vi "Module_ENG_TCPServer.vi"(8 "error in (no error)":errorcluster, 9 "Module ID (-1: Do not Address)":i32=-1, 10 "Wait on Module(s) (\"\": none)":string) -> (0 "error out":errorcluster)   [LabVIEW 2019, in "Module_ENG_TCPServer.lvclass"]
doc: "created using\nJSMA Module Template - ENGINE Class 0.2.1.12\nRob Humfeld - Jet Engineering\nCopyright (c) 2020, Jet Engineering"
uses:
  Module_ENG_TCPServer.lvclass
  <userlib>/Jet Engineering/JET_QSM/Code/Private/JET_QSM - Add State to Front [String API].vi
  Private/Module_ENG_TCPServer_jMsgTxList STYP.ctl
  Private/Module_ENG_TCPServer_jMsgRxList STYP.ctl
  <userlib>/Jet Engineering/JET_QSM/Code/Private/JET_QSM_InvalidOption STYP.ctl
  <userlib>/Jet Engineering/JET_QSM/Code/Private/JET_QSM - Add State [String API].vi
  Private/Module_ENG_TCPServer_EngineStatus STYP.ctl
  Private/Module_ENG_TCPServer_LocalData STYP.ctl
  <userlib>/Jet Engineering/JSMA/Libraries/jMsg_CORE/jMsg_JSMA_ModuleOnline/jMsg_JSMA_ModuleOnline.lvclass
  <userlib>/Jet Engineering/JSMA/Libraries/jMsg_CORE/jMsg_JSMA_ApplicationShutdown/jMsg_JSMA_ApplicationShutdown.lvclass
  <userlib>/Jet Engineering/JSMA/Libraries/jModule Class/jModule.lvclass
  Shared/TCP/jMsgs/jMsg_TCPMessage_Receive/jMsg_TCPMessage_Receive.lvclass
  Shared/TCP/jMsgs/jMsg_TCPMessage_Send/jMsg_TCPMessage_Send.lvclass
  <userlib>/Jet Engineering/JSMA/Libraries/jMsg Class/jMsg.lvclass
  Shared/TCP/jMsgs/jMsg_TCPAcceptor_NewConnection/jMsg_TCPAcceptor_NewConnection.lvclass
  labview_multiplayer_snake_personal/Main Codeline/Software/Code/Shared/TCPReceiver/TCPReceiver.lvclass
  Shared/TCP/TCPPacket/TCPPacket.lvclass
  Shared/TCP/jMsgs/jMsg_TCPServer_Status/jMsg_TCPServer_Status.lvclass
  labview_multiplayer_snake_personal/Main Codeline/Software/Code/Shared/JSONPacket/JSONPacket.lvclass
  C:/Program Files/National Instruments/LabVIEW 2019/user.lib/Jet Engineering/JSMA/Libraries/jModule Class/jModule.lvclass
  C:/projects/labview_multiplayer_snake_personal/Main Codeline/Software/Code/Shared/TCPPacket/TCPPacket.lvclass
  C:/Program Files/National Instruments/LabVIEW 2019/user.lib/Jet Engineering/JSMA/Libraries/jMsg Class/jMsg.lvclass
  <userlib>/Jet Engineering/JSMA/Libraries/jModule Class/Typedefs/jModule_TimerType STYP.ctl
  <userlib>/Jet Engineering/JSMA/Libraries/jModule Class/Typedefs/jModule_TimerConfig STYP.ctl
panel:
  out "Rx jMsg Subscriptions":string[](array[string])
  out "Timer Configuration":T1 {"Expiration Time" format="%<%.3X>T"}
  out "jModule Name":string
  out "iter":i32
  out "Latency, sec.":dbl
  out "RxTime":timestamp format="%<%H:%M:%S%3u>T"
  out "Last Rx Message":string
  out "Recent states before Error (with tick counts)":string
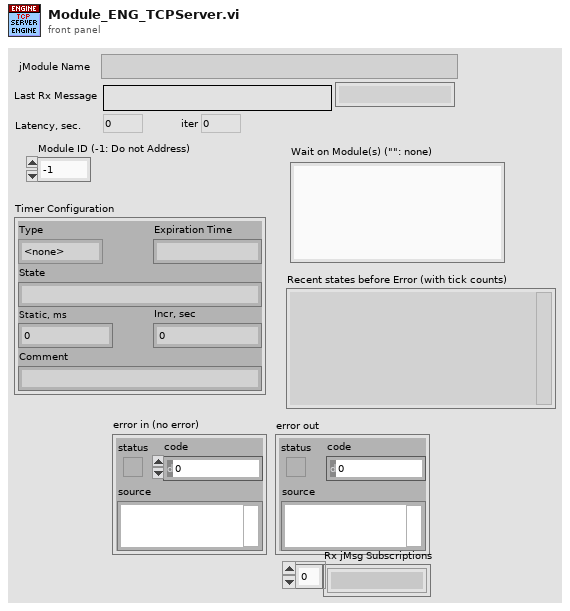
[diagram p1: front panel]
types:
  T1 = typedef "JSMA API.lvlib/jModule.lvclass/jModule_TimerConfig STYP.ctl" = cluster{"Type":T2, "Expiration Time":timestamp, "State":string, "Static, ms":i32, "Incr, sec":dbl, "Comment":string}
  T2 = typedef "JSMA API.lvlib/jModule.lvclass/jModule_TimerType STYP.ctl" = enum16{"<none>", "Static", "Countdown", "Periodic"}
  T3 = typedef "JET_QSM_InvalidOption STYP.ctl" = enum16{"Ignore", "Dialog", "Error"}
  T4 = cluster{"Connection ID":refnum<k5>, "TCPReceiver":refnum<class "TCPReceiver.lvclass">}[]
  T5 = typedef "Module_ENG_TCPServer.lvclass/Module_ENG_TCPServer_LocalData STYP.ctl" = cluster{"VI":cluster{"error":errorcluster, "isExiting?":bool}, "EngineStatus":T6}
  T6 = typedef "Module_ENG_TCPServer.lvclass/Module_ENG_TCPServer_EngineStatus STYP.ctl" = cluster{"Connections":cluster{"Connection ID":refnum<k5>, "TCPReceiver":refnum<class "TCPReceiver.lvclass">}[]}
  T7 = typedef "Module_ENG_TCPServer.lvclass/Module_ENG_TCPServer_jMsgRxList STYP.ctl" = cluster{"<placeholder>":refnum<class "jMsg_JSMA_ApplicationShutdown.lvclass">, "jMsg_TCPMessage_Send":refnum<class "jMsg_TCPMessage_Send.lvclass">, "jMsg_TCPAcceptor_NewConnection":refnum<class "jMsg_TCPAcceptor_NewConnection.lvclass">}
  T8 = typedef "Module_ENG_TCPServer.lvclass/Module_ENG_TCPServer_jMsgTxList STYP.ctl" = cluster{"<placeholder>":refnum<class "jMsg_JSMA_ModuleOnline.lvclass">, "jMsg_TCPMessage_Receive":refnum<class "jMsg_TCPMessage_Receive.lvclass">, "jMsg_TCPServer_Status":refnum<class "jMsg_TCPServer_Status.lvclass">}
  T9 = typedef "JET_QSM_Refnum STYP.ctl" = cluster{"state":cluster{"queue":refnum<queue>, "idle":string, "error":string, "STOP":string}, "debug":cluster{"enabled?":bool, "queue":refnum<queue>}, "Invalid.option":T3, "QSM.Name":string}
  T10 = typedef "JET_QSM_Element STYP.ctl" = cluster{"state":string, "data":variant, "comment":string}
  T11 = cluster{"Connection ID":refnum<k5>, "TCPReceiver out":refnum<class "TCPReceiver.lvclass">}
  T12 = cluster{"Connection ID":refnum<k5>, "TCPReceiver out":refnum<class "TCPReceiver.lvclass">}[]
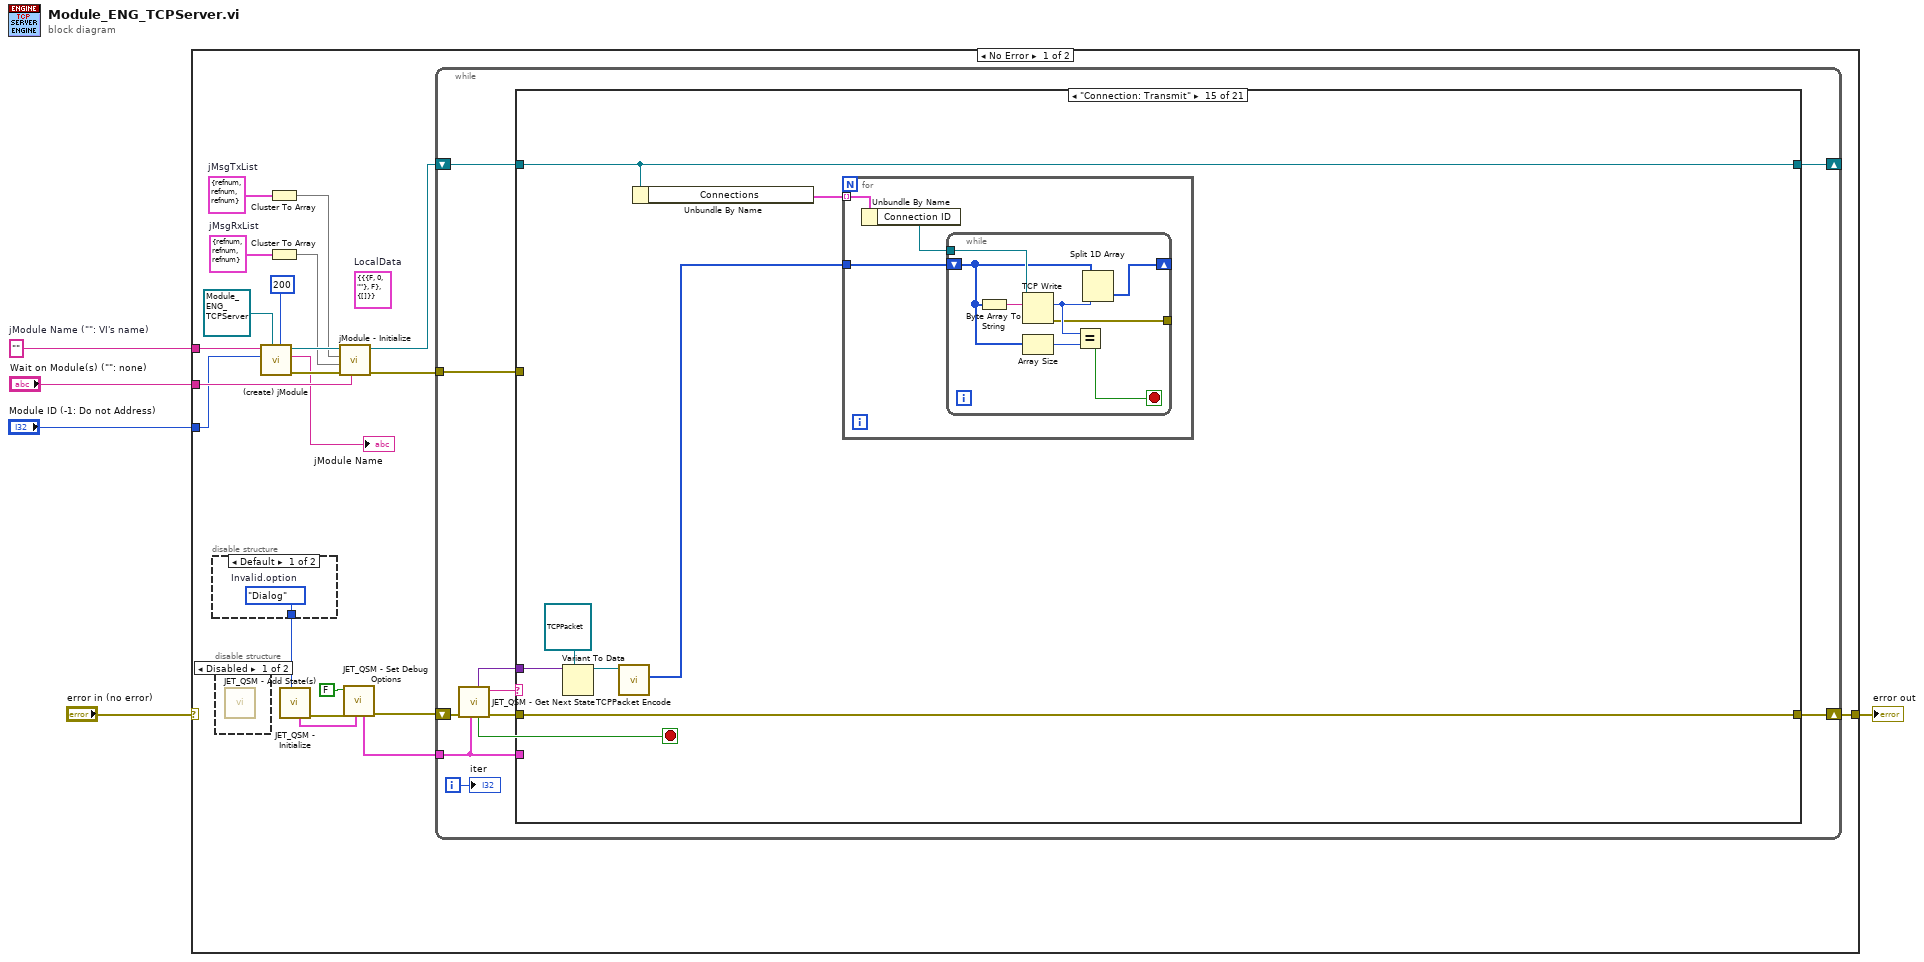
[diagram p0: block diagram]
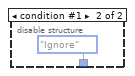
[diagram p3: hidden frame]
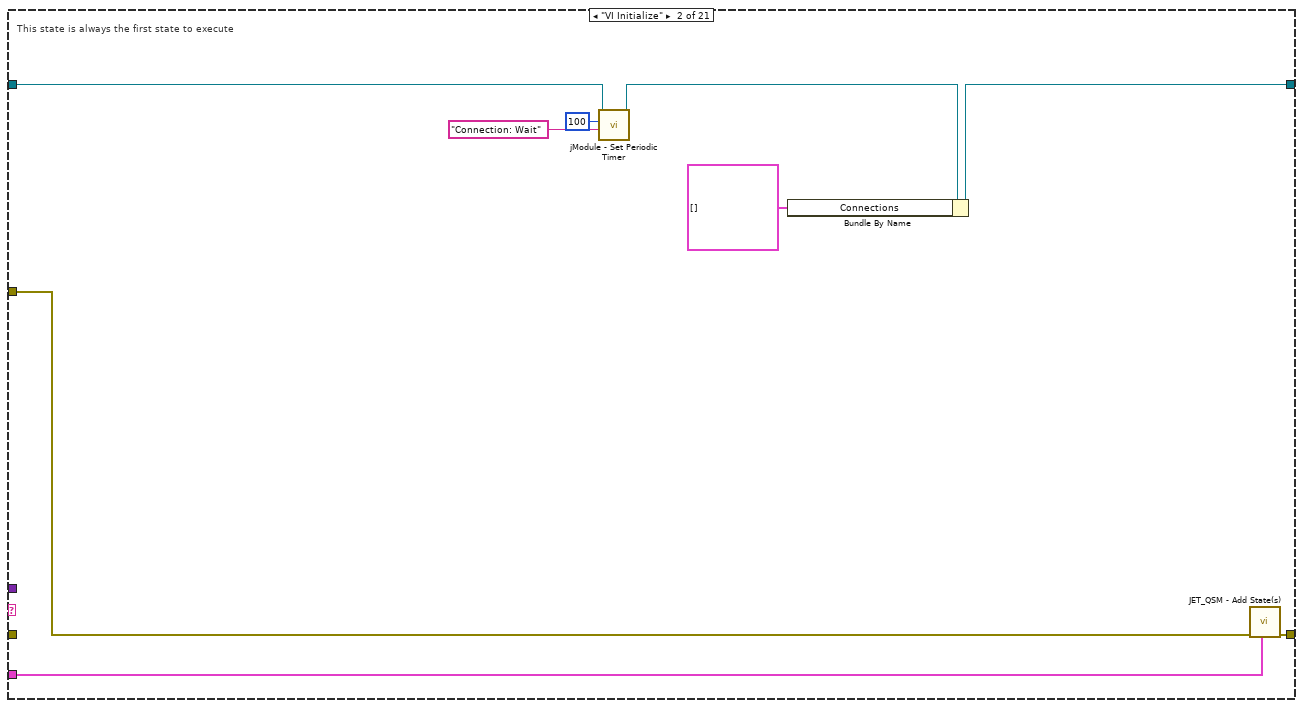
[diagram p5: hidden frame]
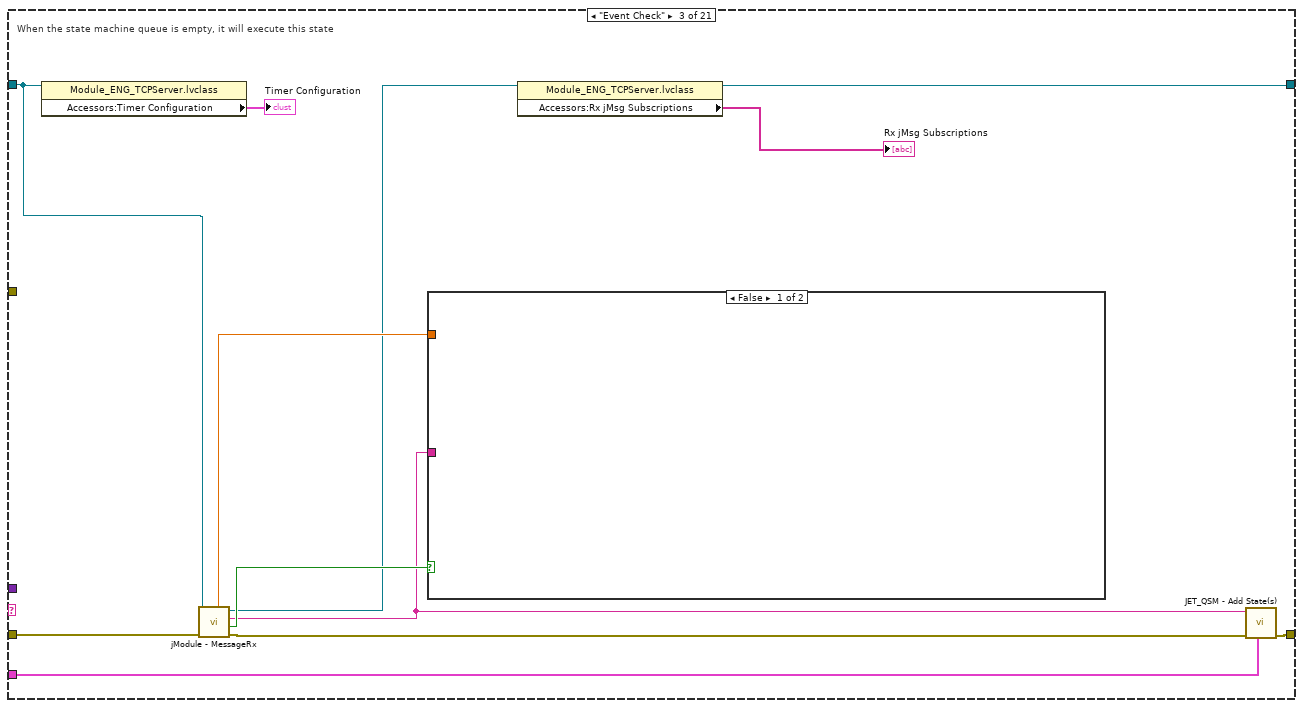
[diagram p6: hidden frame]
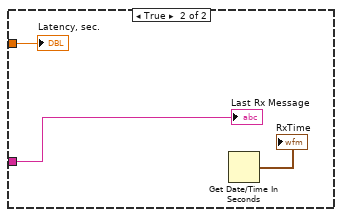
[diagram p7: hidden frame]
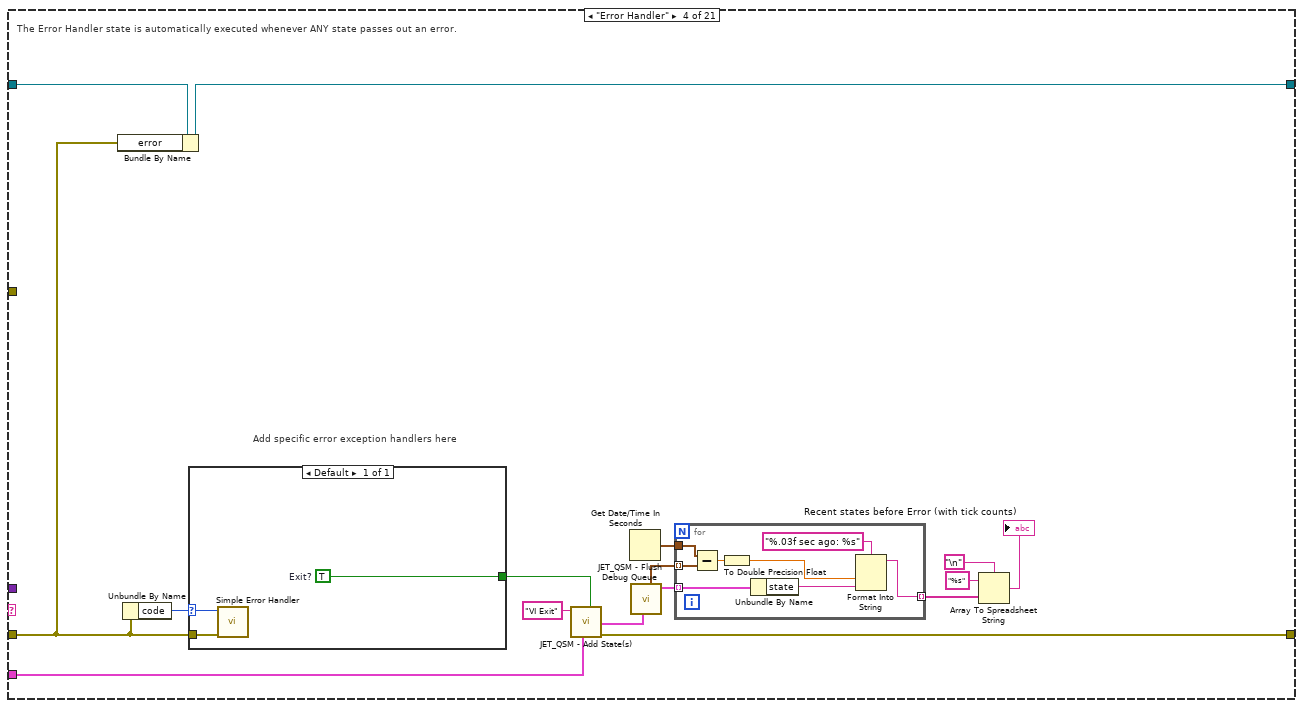
[diagram p8: hidden frame]
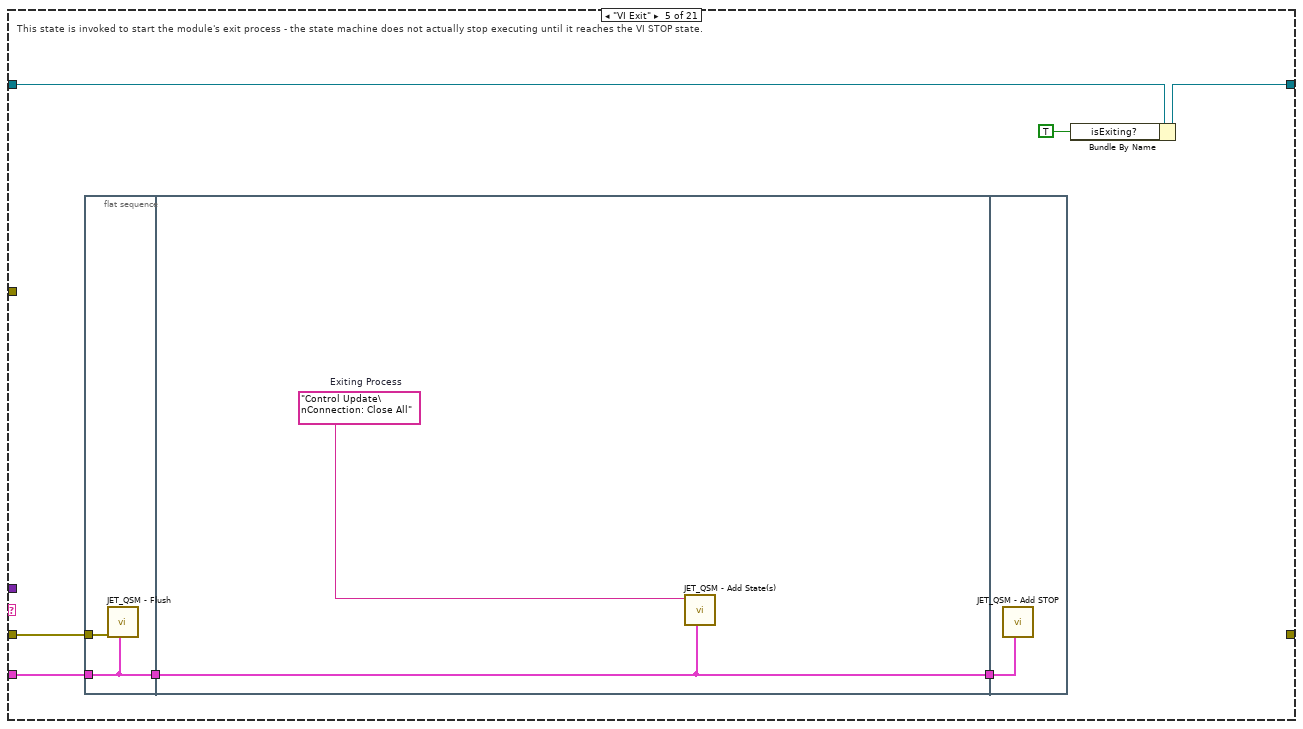
[diagram p9: hidden frame]
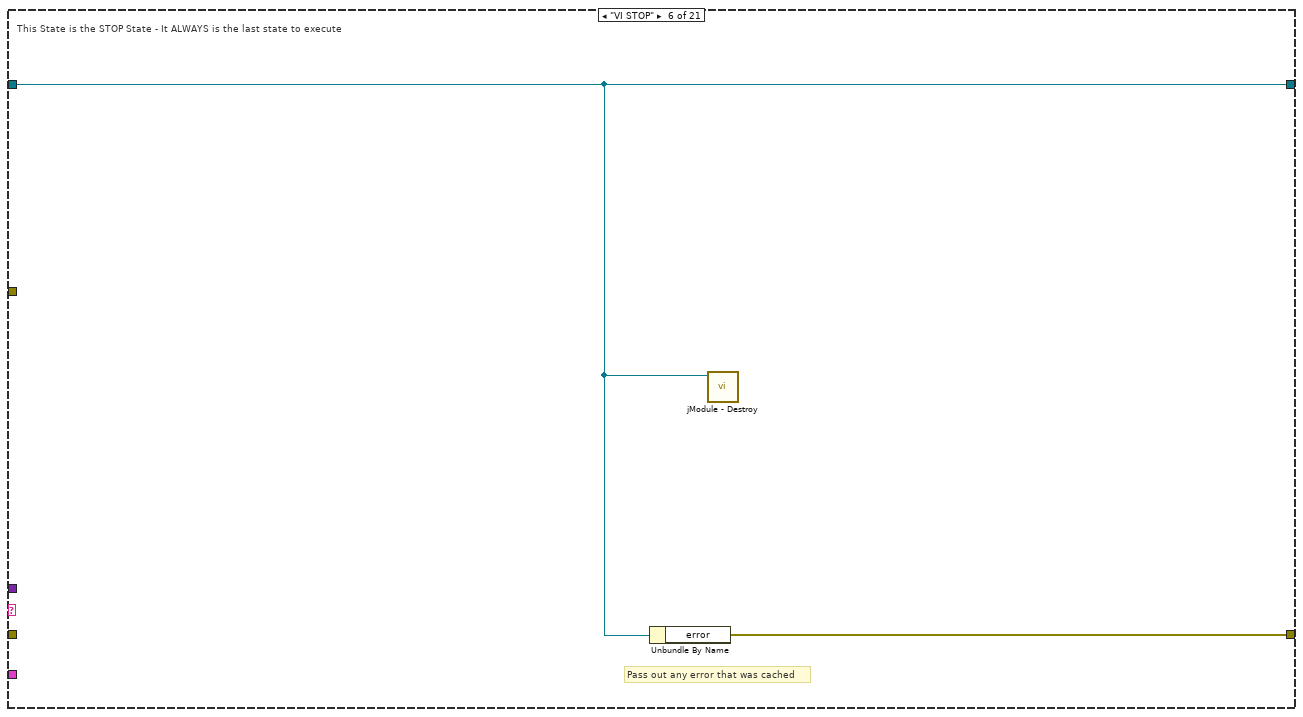
[diagram p10: hidden frame]
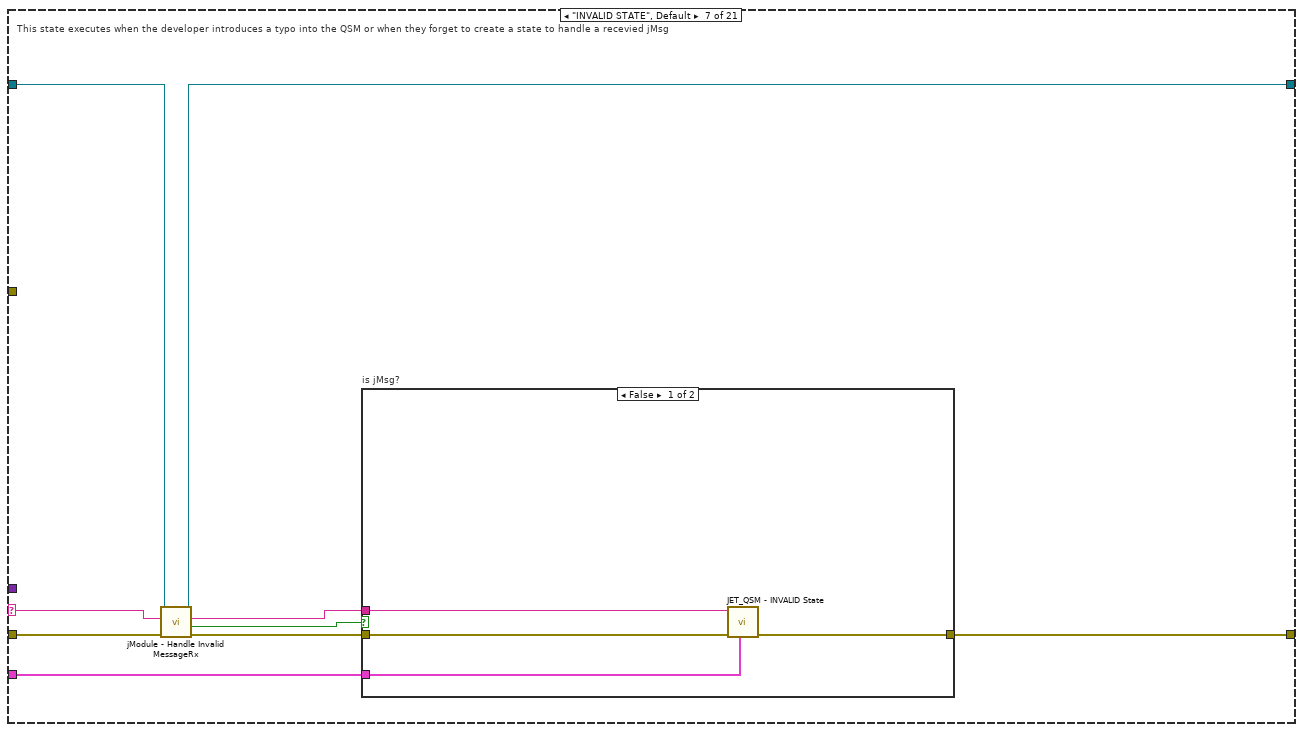
[diagram p11: hidden frame]
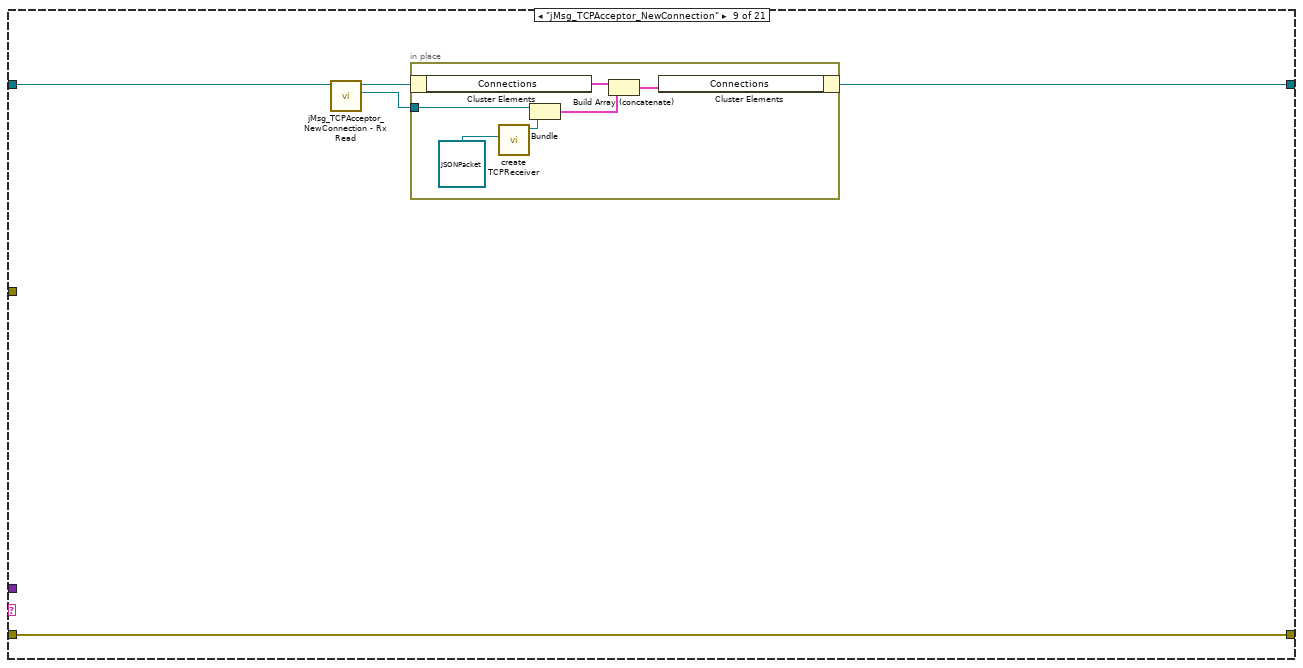
[diagram p14: hidden frame]
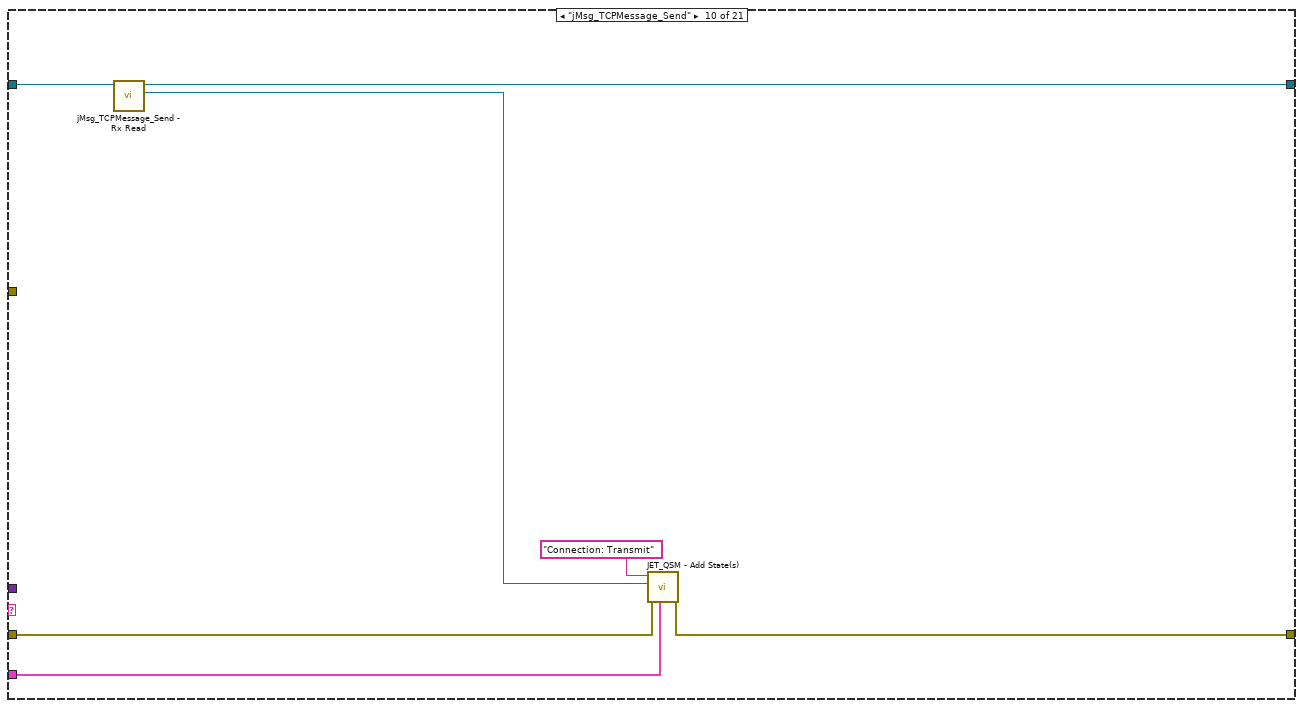
[diagram p15: hidden frame]
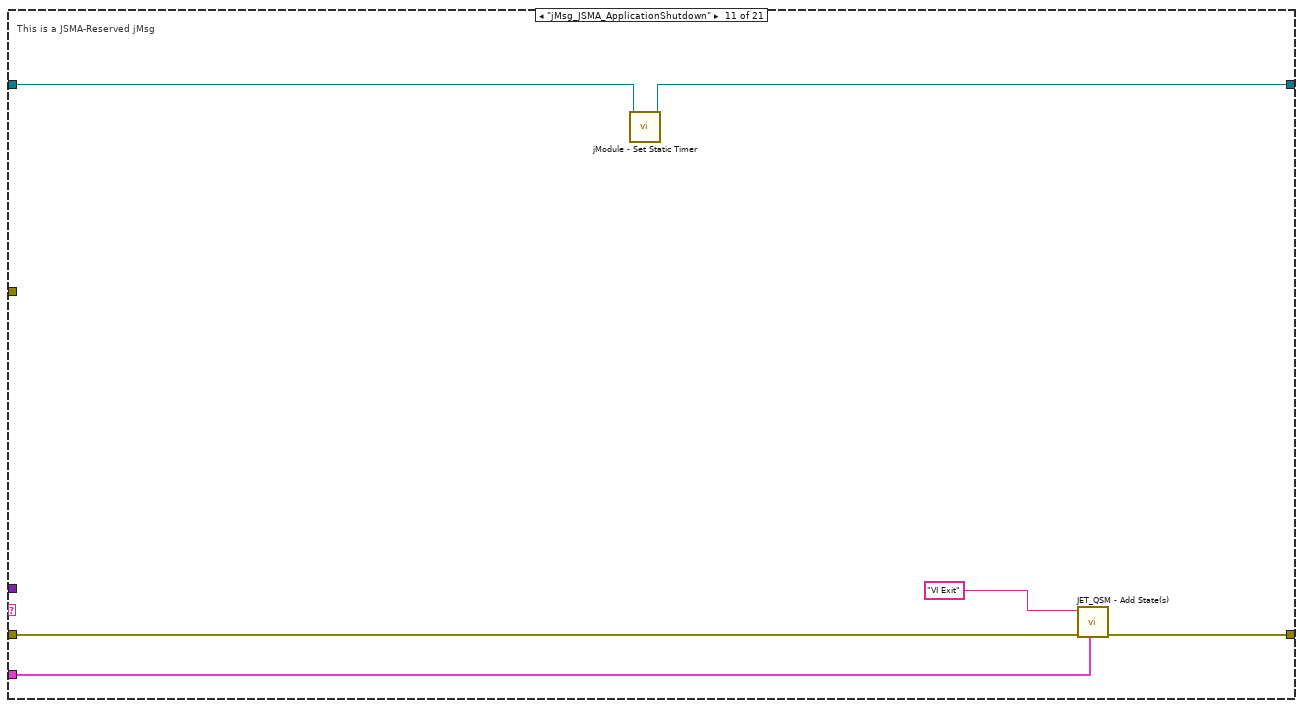
[diagram p16: hidden frame]
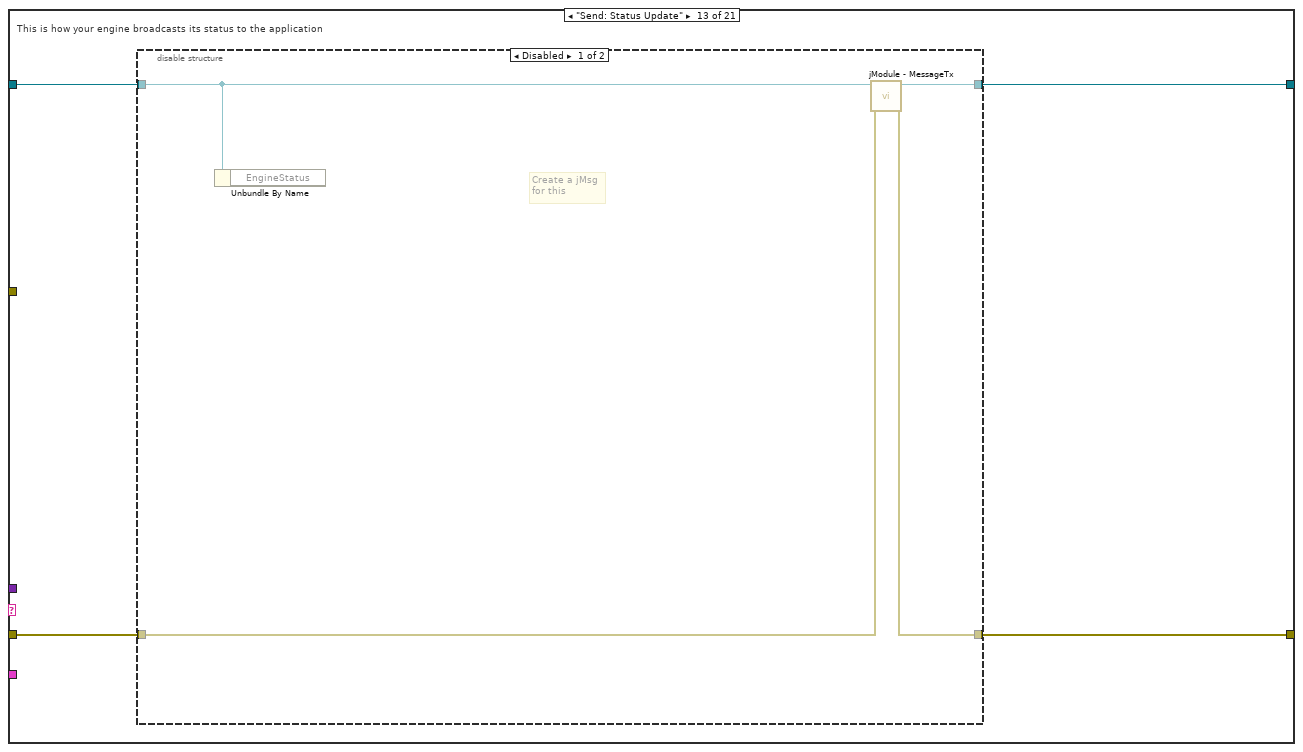
[diagram p18: hidden frame]
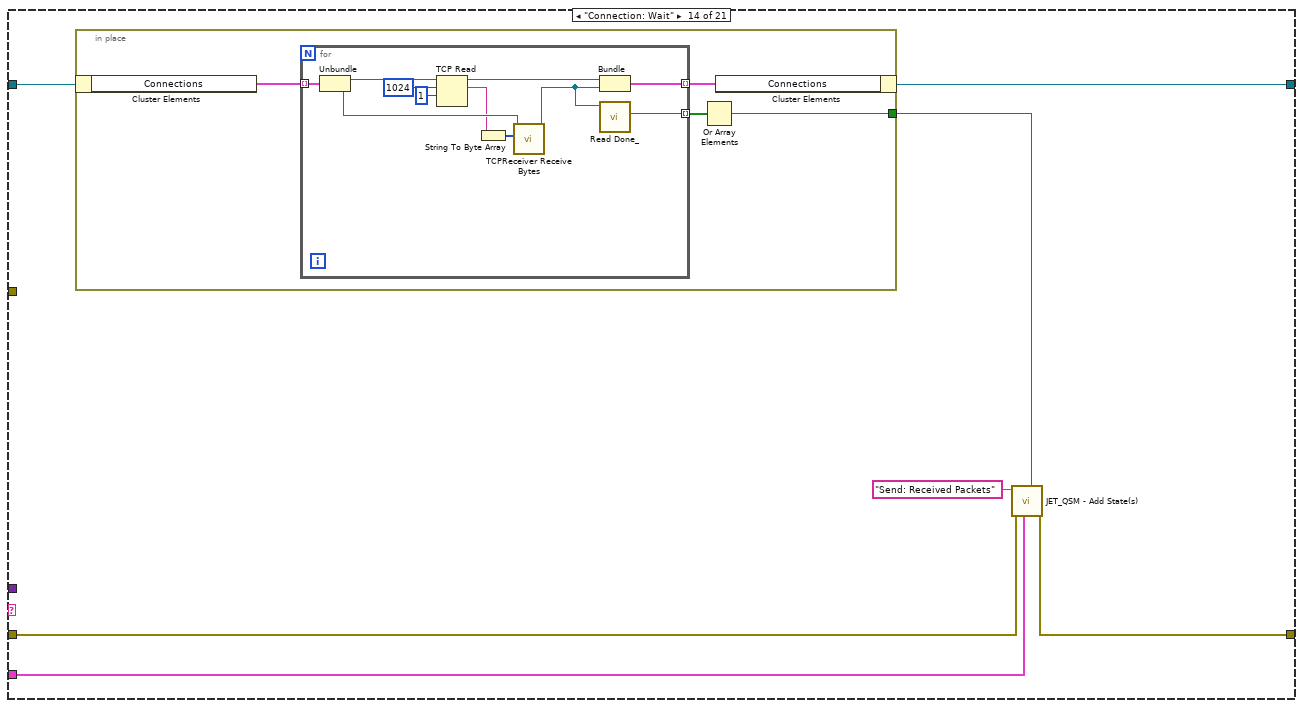
[diagram p20: hidden frame]
diagram:
  w3 = ""  # jModule Name ("": VI's name)
  n1 = case shown="No Error" "error in (no error)" {
    selector: "error in (no error)" -> [_ w238]
    tunnel: [w10 w238] -> w5
    tunnel: "Wait on Module(s) (\"\": none)" -> [w17 _]
    tunnel: w3 -> [w16 _]
    tunnel: "Module ID (-1: Do not Address)" -> [w9 _]
    frame No Error {
      (unwired) T5 {"VI"={"error"={"status"=FALSE, "code"=0, "source"=""}, "isExiting?"=FALSE}, "EngineStatus"={"Connections"=[]}}  # LocalData
      w14 = T7 {"<placeholder>"=refnum, "jMsg_TCPMessage_Send"=refnum, "jMsg_TCPAcceptor_NewConnection"=refnum}  # jMsgRxList
      w15 = T8 {"<placeholder>"=refnum, "jMsg_TCPMessage_Receive"=refnum, "jMsg_TCPServer_Status"=refnum}  # jMsgTxList
      n2 = disable-structure shown="Default" {
        disable-tunnel: [w27 JET_QSM_InvalidOption_STYP."Ignore" ("Invalid.option (Dialog)")] -> w18
        frame condition #0 (active) {
          w27 = JET_QSM_InvalidOption_STYP."Dialog"  # Invalid.option
        }
        frame condition #1 {
        }
      }
      n3 = disable-structure shown="Disabled" {
        frame Disabled {
          n4 = call-poly <userlib>:"JET_QSM - Add State(s).vi"() -> ()  [unwired: 11 in, 1 out]
        }
        frame Enabled {
        }
      }
      n5 = call <userlib>:"(create) jModule.vi"("Max Queue size (50)"=200, "jModule Child class"=refnum<class "Module_ENG_TCPServer.lvclass"> refnum ("jModule Template_ENGINEClass.lvclass"), "Module ID (-1: Do Not Address)"=w9, "jModule Name (\"\": use calling VI's name)"=w16) -> ("error out"=w19:errorcluster, "jModule Name"=→"jModule Name":string, "jModule"=w22:refnum<class "Module_ENG_TCPServer.lvclass">)  [unwired: 4 in, 1 out]
      n6 = Cluster To Array(cluster=w15) -> (array=w21:refnum<class "jMsg.lvclass">[])
      n7 = Cluster To Array(cluster=w14) -> (array=w20:refnum<class "jMsg.lvclass">[])
      n8 = call <userlib>:"JET_QSM - Initialize.vi"("invalid state action (Dialog)"=w18) -> ("error out"=w23:errorcluster, "Jet_QSM refnum"=w25:T9)  [unwired: 9 in]
      n9 = call-dynamic "jModule - Initialize.vi"("Wait on Module(s) (\"\": none)"=w17, "error in (no error)"=w19, "jMsgRxList"=w20, "jMsgTxList"=w21, "jModule"=w22) -> ("error out"=w11:errorcluster, "jModule"=w6:refnum<class "Module_ENG_TCPServer.lvclass">)  [unwired: 5 in]
      n10 = call <userlib>:"JET_QSM - Set Debug Options.vi"("Jet_QSM refnum"=w25, "error in (no error)"=w23, "debug.enabled? (F)"=FALSE) -> ("error out"=w12:errorcluster, "Jet_QSM ref"=w24:T9)  [unwired: 7 in]
      n11 = while {
        tunnel: w24 -> [w30]
        shift-right: [w34] -> _
        shift-left: w6 -> [w35]
        shift-right: [w33] -> w10
        shift-left: w12 -> [w39]
        tunnel: w11 -> [w31]
        i -> [w32]
        stop <- w36 stop-if-true
        n12 = call <userlib>:"JET_QSM - Get Next State.vi"("Jet_QSM refnum"=w30, "error in (no error)"=w39) -> ("error out"=w38:errorcluster, "state"=w37:string, "Stop Loop?"=w36:bool, "state data"=w29:variant)  [unwired: 5 in, 1 out]
        n13 = case shown="\"Connection: Transmit\"" w37 {
          selector: w37 -> [_ _ _ _ _ _ w110 _ _ _ _ _ _ _ _ _ _ _ _ _ _]
          tunnel: w38 -> [w40 _ w60 w70 w98 _ w111 w120 w126 w136 w142 w146 w150 w161 w186 w198 w202 w209 w229 w231 w236]
          tunnel: w35 -> [w41 w46 w56 w67 w93 w105 w107 w121 w125 w138 w140 w147 w148 w163 w183 w199 w201 w208 w230 w232 w237]
          tunnel: [w41 w43 w52 w66 w92 w105 w106 w121 w123 w139 w141 w147 w151 w164 w183 w199 w201 w205 w230 w232 w237] -> w34
          tunnel: [w40 w50 w61 w73 _ w104 w109 w120 w126 w137 w144 w146 w149 w162 w186 w198 w202 w209 w229 w234 w236] -> w33
          tunnel: w31 -> [_ w48 _ _ _ _ _ _ _ _ _ _ _ _ _ _ _ _ _ _ _]
          tunnel: w30 -> [_ w49 w62 w72 w97 _ w108 _ _ w135 w145 _ _ w160 _ _ _ _ _ w235 _]
          tunnel: w29 -> [_ _ _ _ _ _ _ _ _ _ _ _ _ _ w185 _ _ _ _ _ _]
          frame "------ Standard States ------" {
            # "Standard States are required states for a JET_QSM State Machine\n\nTheir names may be changed; use the Initialize function to specify the new names"
            # "This is a section header; the state is never expected to execute"
          }
          frame "VI Initialize" {
            # "This state is always the first state to execute"
            n14 = call <userlib>:"jModule - Set Periodic Timer.vi"("Go to State Periodically (\"\": no change)"="Connection: Wait" ("Go to State Periodically (\"\": no change)"), "Timing Period, ms"=u32 100, "jModule"=w46) -> ("jModule"=w47:refnum<class "Module_ENG_TCPServer.lvclass">)  [unwired: 7 in, 1 out]
            n15 = Bundle By Name(cluster=w47, "Connections"=T4 [] ("My.EngineStatus.Connections")) -> (w43:refnum<class "Module_ENG_TCPServer.lvclass">)
            n16 = call-poly <userlib>:"JET_QSM - Add State(s).vi"("Jet_QSM refnum"=w49, "error in (no error)"=w48) -> ("error out"=w50:errorcluster)  [unwired: 9 in]
          }
          frame "Event Check" {
            # "When the state machine queue is empty, it will execute this state"
            n17 = property class="Module_ENG_TCPServer.lvclass"(reference=w56) -> ("Accessors:Timer Configuration"=→"Timer Configuration":T1)  [unwired: 1 in, 2 out]
            n18 = call-dynamic "jModule - MessageRx.vi"("error in (no error)"=w60, "jModule"=w56) -> ("error out"=w55:errorcluster, "MsgRx?"=w59:bool, "QSMState"=w57:string, "jModule"=w54:refnum<class "Module_ENG_TCPServer.lvclass">, "Latency, sec."=w58:dbl)  [unwired: 4 in, 1 out]
            n19 = case shown="False" w59 {
              tunnel: w57 -> [_ w64]
              tunnel: w58 -> [_ w65]
              frame False {
              }
              frame True {
                n20 = Get Date/Time In Seconds() -> (seconds since 1Jan1904=→"RxTime":timestamp)
                "Last Rx Message" <- w64
                "Latency, sec." <- w65
              }
            }
            n21 = property class="Module_ENG_TCPServer.lvclass"(reference=w54) -> (reference out=w52:refnum<class "Module_ENG_TCPServer.lvclass">, "Accessors:Rx jMsg Subscriptions"=→"Rx jMsg Subscriptions":string[])  [unwired: 1 in, 1 out]
            n22 = call-poly <userlib>:"JET_QSM - Add State(s).vi"("Jet_QSM refnum"=w62, "error in (no error)"=w55, "state(s)"=w57) -> ("error out"=w61:errorcluster)  [unwired: 8 in]
          }
          frame "Error Handler" {
            # "Add specific error exception handlers here"
            # "The Error Handler state is automatically executed whenever ANY state passes out an error."
            n23 = Bundle By Name(cluster=w67, "error"=w70) -> (w66:refnum<class "Module_ENG_TCPServer.lvclass">)
            n24 = Unbundle By Name(w70) -> ("code"=w68:i32)
            n25 = case shown="Default" w68 {
              selector: w68 -> [w82]
              tunnel: [w83] -> w69
              tunnel: w70 -> [w81]
              frame Default {
                w83 = TRUE  # Exit?
                n26 = call <vilib>:"Simple Error Handler.vi"("error code (no error:0)"=w82, "error in (no error)"=w81) -> ()  [unwired: 3 in, 5 out]
              }
            }
            n27 = call-poly <userlib>:"JET_QSM - Add State(s).vi"("act? (T)"=w69, "Jet_QSM refnum"=w72, "state(s)"="VI Exit") -> ("error out"=w73:errorcluster)  [unwired: 8 in]
            n28 = Get Date/Time In Seconds() -> (seconds since 1Jan1904=w76:timestamp)
            n29 = call <userlib>:"JET_QSM - Flush Debug Queue.vi"("Jet_QSM refnum"=w72) -> ("QSM Elements"=w74:T10[], "Timestamps"=w75:timestamp[])  [unwired: 8 in, 1 out]
            n30 = for {
              tunnel: w74 -> [w91] mode=indexing
              tunnel: [w89] -> w78 mode=indexing
              tunnel: w76 -> [w86]
              tunnel: w75 -> [w87] mode=indexing
              n31 = Subtract(x=w86, y=w87) -> (x-y=w85:dbl)
              n32 = To Double Precision Float(number=w85) -> (double precision float=w84:dbl)
              n33 = Unbundle By Name(w91) -> ("state"=w90:string)
              n34 = Format Into String(format string="%.03f sec ago: %s", w84, w90) -> (resulting string=w89:string)  [unwired: 2 in, 1 out]
            }
            n35 = Array To Spreadsheet String(delimiter (Tab)="\n", array=w78, 3:"%s" ("format string")) -> (spreadsheet string=→"Recent states before Error (with tick counts)":string)
          }
          frame "VI Exit" {
            # "This state is invoked to start the module's exit process - the state machine does not actually stop executing until it reaches the VI STOP state."
            n36 = flat-sequence {
              tunnel: w98 -> [w100]
              tunnel: w97 -> [w99]
              tunnel: [w99] -> w96
              tunnel: w96 -> [w102]
              tunnel: [w102] -> w95
              tunnel: w95 -> [w103]
              frame #0 {
                n37 = call <userlib>:"JET_QSM - Flush.vi"("Jet_QSM ref"=w99, "error in (no error)"=w100) -> ()  [unwired: 8 in, 2 out]
              }
              frame #1 {
                w101 = "Control Update\nConnection: Close All"  # Exiting Process
                n38 = call-poly <userlib>:"JET_QSM - Add State(s).vi"("Jet_QSM refnum"=w102, "state(s)"=w101) -> ()  [unwired: 9 in, 1 out]
              }
              frame #2 {
                n39 = call <userlib>:"JET_QSM - Add STOP.vi"("Jet_QSM refnum"=w103) -> ()  [unwired: 10 in, 1 out]
              }
            }
            n40 = Bundle By Name(cluster=w93, "isExiting?"=TRUE ("VI.isExiting?")) -> (w92:refnum<class "Module_ENG_TCPServer.lvclass">)
          }
          frame "VI STOP" {
            # "Pass out any error that was cached"
            # "This State is the STOP State - It ALWAYS is the last state to execute"
            n41 = Unbundle By Name(w105) -> ("error"=w104:errorcluster)
            n42 = call-dynamic "jModule - Destroy.vi"("jModule"=w105) -> ()  [unwired: 10 in, 1 out]
          }
          frame "INVALID STATE", Default {
            # "This state executes when the developer introduces a typo into the QSM or when they forget to create a state to handle a recevied jMsg"
            n43 = call-dynamic "jModule - Handle Invalid MessageRx.vi"("error in (no error)"=w111, "Invalid State"=w110, "jModule"=w107) -> ("error out"=w114:errorcluster, "is jMsg State?"=w112:bool, "Invalid State"=w113:string, "jModule"=w106:refnum<class "Module_ENG_TCPServer.lvclass">)  [unwired: 5 in]
            n44 = case "is jMsg?" shown="False" w112 {
              tunnel: w108 -> [w116 _]
              tunnel: [w115 w119] -> w109
              tunnel: w114 -> [w117 w119]
              tunnel: w113 -> [w118 _]
              frame False {
                n45 = call <userlib>:"JET_QSM - INVALID State.vi"("Jet_QSM refnum"=w116, "error in (no error)"=w117, "state"=w118) -> ("error out"=w115:errorcluster)  [unwired: 8 in]
              }
              frame True {
              }
            }
          }
          frame "------ jMsg  ------" {
            # "This is a section header; the state is never expected to execute"
          }
          frame "jMsg_TCPAcceptor_NewConnection" {
            n46 = call "jMsg_TCPAcceptor_NewConnection - Rx Read.vi"("jModule"=w125) -> ("Connection ID"=w122:refnum<k5>, "jModule"=w124:refnum<class "Module_ENG_TCPServer.lvclass">)  [unwired: 7 in, 2 out]
            n47 = in-place {
              in-place-border: w122 -> [w130]
              n48 = in-place-cluster #1(w124) -> ("Connections"=w132:T4)
              n49 = call "create TCPReceiver.vi"("Packet Type"=refnum<class "JSONPacket.lvclass"> refnum ("JSONPacket.lvclass")) -> ("TCPReceiver out"=w128:refnum<class "TCPReceiver.lvclass">)  [unwired: 9 in, 1 out]
              n50 = Bundle("Connection ID"=w130, "TCPReceiver out"=w128) -> (w129:T11)  [unwired: 1 in]
              n51 = Build Array (concatenate)(w132, w129) -> (w131:T12)
              n52 = in-place-cluster #1("Connections"=w131) -> (w123:refnum<class "Module_ENG_TCPServer.lvclass">)
            }
          }
          frame "jMsg_TCPMessage_Send" {
            n53 = call "jMsg_TCPMessage_Send - Rx Read.vi"("jModule"=w138) -> ("TCPPacket"=w133:refnum<class "TCPPacket.lvclass">, "jModule"=w139:refnum<class "Module_ENG_TCPServer.lvclass">)  [unwired: 7 in, 2 out]
            n54 = call-poly <userlib>:"JET_QSM - Add State(s).vi"("Jet_QSM refnum"=w135, "error in (no error)"=w136, "state(s) data [ALL states]"=w133, "state(s)"="Connection: Transmit") -> ("error out"=w137:errorcluster)  [unwired: 7 in]
          }
          frame "jMsg_JSMA_ApplicationShutdown" {
            # "This is a JSMA-Reserved jMsg"
            n55 = call <userlib>:"jModule - Set Static Timer.vi"("jModule"=w140) -> ("jModule"=w141:refnum<class "Module_ENG_TCPServer.lvclass">)  [unwired: 9 in, 1 out]
            n56 = call-poly <userlib>:"JET_QSM - Add State(s).vi"("Jet_QSM refnum"=w145, "error in (no error)"=w142, "state(s)"="VI Exit") -> ("error out"=w144:errorcluster)  [unwired: 8 in]
          }
          frame "------ Actions  ------" {
            # "This is a section header; the state is never expected to execute"
          }
          frame "Send: Status Update" {
            # "This is how your engine broadcasts its status to the application"
            n57 = disable-structure shown="Disabled" {
              disable-tunnel: [w154 w157] -> w151
              disable-tunnel: w150 -> [w153 w156]
              disable-tunnel: [w152 w156] -> w149
              disable-tunnel: w148 -> [w155 w157]
              frame Disabled {
                # "Create a jMsg\nfor this"
                n58 = Unbundle By Name(w155) -> ()  [unwired: 1 out]
                n59 = call <userlib>:"jModule - MessageTx.vi"("error in (no error)"=w153, "jModule"=w155) -> ("error out"=w152:errorcluster, "jModule"=w154:refnum<class "Module_ENG_TCPServer.lvclass">)  [unwired: 6 in, 2 out]
              }
              frame Enabled {
              }
            }
          }
          frame "Connection: Wait" {
            n60 = in-place {
              in-place-border: [w165] -> w158
              n61 = in-place-cluster #2(w163) -> ("Connections"=w168:T4)
              n62 = for {
                tunnel: w168 -> [w179] mode=indexing
                tunnel: [w172] -> w167 mode=indexing
                tunnel: [w170] -> w166 mode=indexing
                n63 = Unbundle(w179) -> ("Connection ID"=w178:refnum<k5>, "TCPReceiver"=w177:refnum<class "TCPReceiver.lvclass">)
                n64 = TCP Read(connection ID=w178, bytes to read=1024, 9:1 ("timeout ms (25000)")) -> (connection ID out=w173:refnum<k5>, data out=w175:string)  [unwired: 2 in, 1 out]
                n65 = String To Byte Array(string=w175) -> (unsigned byte array=w176:u8[])
                n66 = call-dynamic "TCPReceiver Receive Bytes.vi"("Data"=w176, "TCPReceiver in"=w177) -> ("TCPReceiver out"=w171:refnum<class "TCPReceiver.lvclass">)  [unwired: 8 in, 1 out]
                n67 = Bundle("Connection ID"=w173, "TCPReceiver out"=w171) -> (w172:T11)  [unwired: 1 in]
                n68 = call-dynamic "Read Done_.vi"("TCPReceiver in"=w171) -> ("Done?"=w170:bool)  [unwired: 8 in, 2 out]
              }
              n69 = Or Array Elements(Boolean array=w166) -> (logical OR=w165:bool)
              n70 = in-place-cluster #2("Connections"=w167) -> (w164:refnum<class "Module_ENG_TCPServer.lvclass">)
            }
            n71 = call-poly <userlib>:"JET_QSM - Add State(s).vi"("act? (T)"=w158, "Jet_QSM refnum"=w160, "error in (no error)"=w161, "state(s)"="Send: Received Packets") -> ("error out"=w162:errorcluster)  [unwired: 7 in]
          }
          frame "Connection: Transmit" {
            n72 = Variant To Data(type=refnum<class "TCPPacket.lvclass"> refnum ("TCPPacket.lvclass"), Variant=w185) -> (data=w181:refnum<class "TCPPacket.lvclass">)  [unwired: 1 in, 1 out]
            n73 = call-dynamic "TCPPacket Encode.vi"("TCPPacket in"=w181) -> ("Data"=w180:u8[])  [unwired: 8 in, 2 out]
            n74 = Unbundle By Name(w183) -> ("Connections"=w182:T4)
            n75 = for {
              tunnel: w182 -> [w189] mode=indexing
              tunnel: w180 -> [w187]
              n76 = Unbundle By Name(w189) -> ("Connection ID"=w188:refnum<k5>)
              n77 = while {
                tunnel: w188 -> [w197]
                shift-right: [w195] -> _
                shift-left: w187 -> [w194]
                tunnel: [w190] -> _
                stop <- w191 stop-if-true
                n78 = Byte Array To String(unsigned byte array=w194) -> (string=w196:string)
                n79 = TCP Write(connection ID=w197, data in=w196) -> (bytes written=w192:i32, error out=w190:errorcluster)  [unwired: 2 in, 1 out]
                n80 = Array Size(array=w194) -> (size(s)=w193:i32)
                n81 = Equal?(x=w192, y=w193) -> (x = y?=w191:bool)
                n82 = Split 1D Array(array=w194, index=w192) -> (second subarray=w195:u8[])  [unwired: 1 out]
              }
            }
          }
          frame "Connection: Close" {
          }
          frame "Connection: Close All" {
            n83 = Unbundle By Name(w201) -> ("Connections"=w200:T4)
            n84 = for {
              tunnel: w200 -> [w204] mode=indexing
              n85 = Unbundle(w204) -> ("Connection ID"=w203:refnum<k5>)  [unwired: 1 out]
              n86 = TCP Close Connection(connection ID=w203) -> ()  [unwired: 2 in, 2 out]
            }
          }
          frame "Send: Received Packets" {
            n87 = in-place {
              in-place-border: [w214] -> w207
              n88 = in-place-cluster #3(w208) -> ("Connections"=w216:T4)
              n89 = for {
                tunnel: w216 -> [w223] mode=indexing
                tunnel: [w221] -> w214 mode=indexing if=w220
                tunnel: [w217] -> w215 mode=indexing
                n90 = Unbundle(w223) -> ("Connection ID"=w218:refnum<k5>, "TCPReceiver"=w222:refnum<class "TCPReceiver.lvclass">)
                n91 = call-dynamic "Read Done_.vi"("TCPReceiver in"=w222) -> ("Done?"=w220:bool)  [unwired: 8 in, 2 out]
                n92 = case shown="True" w220 {
                  tunnel: w222 -> [w224 w228]
                  tunnel: [w224 w226] -> w219
                  tunnel: [_ w225] -> w221
                  frame False {
                  }
                  frame True {
                    n93 = call-dynamic "Read Packet.vi"("TCPReceiver in"=w228) -> ("TCPPacket.lvclass"=w225:refnum<class "TCPPacket.lvclass">, "TCPReceiver out"=w227:refnum<class "TCPReceiver.lvclass">)  [unwired: 8 in, 1 out]
                    n94 = call-dynamic "TCPReceiver Reset.vi"("TCPReceiver in"=w227) -> ("TCPReceiver out"=w226:refnum<class "TCPReceiver.lvclass">)  [unwired: 9 in, 1 out]
                  }
                }
                n95 = Bundle("Connection ID"=w218, "TCPReceiver out"=w219) -> (w217:T11)  [unwired: 1 in]
              }
              n96 = in-place-cluster #3("Connections"=w215) -> (w206:refnum<class "Module_ENG_TCPServer.lvclass">)
            }
            n97 = for {
              tunnel: w207 -> [w210] mode=indexing
              shift-right: [w212] -> w205
              shift-left: w206 -> [w213]
              n98 = call "jMsg_TCPMessage_Receive (create).vi"("Packet"=w210) -> ("jMsg_TCPMessage_Receive"=w211:refnum<class "jMsg_TCPMessage_Receive.lvclass">)  [unwired: 9 in, 1 out]
              n99 = call <userlib>:"jModule - MessageTx.vi"("jMsg"=w211, "jModule"=w213) -> ("jModule"=w212:refnum<class "Module_ENG_TCPServer.lvclass">)  [unwired: 6 in, 3 out]
            }
          }
          frame "------ Window and Panel Control ------" {
            # "This is a section header; the state is never expected to execute"
          }
          frame "Control Update" {
            # "Update all control properties values from the status cluster in this state - in this way we can separate the View from the Model and Controller, as well as consolidate/reduce locals and property nodes"
            n100 = call-poly <userlib>:"JET_QSM - Add State(s).vi"("Jet_QSM refnum"=w235, "error in (no error)"=w231, "state(s)"="Indicator Update") -> ("error out"=w234:errorcluster)  [unwired: 8 in]
          }
          frame "Indicator Update" {
            # "Update all indicator properties and values from the status cluster in this state - in this way we can separate the View from the Model and Controller, as well as consolidate/reduce property nodes"
          }
        }
        "iter" <- w32
      }
    }
    frame Error {
    }
  }
  "error out" <- w5
